vi "GEA3_Tool (Main).vi"() -> ()   [LabVIEW 2021]
panel:
  in  "Numeric":u64 format="%x"
  out "substring":string
  in  "dato":string="F039"
  in  "Write":bool
  in  "Read":bool
  in  "stop":bool
  out "CompleteFrame":string
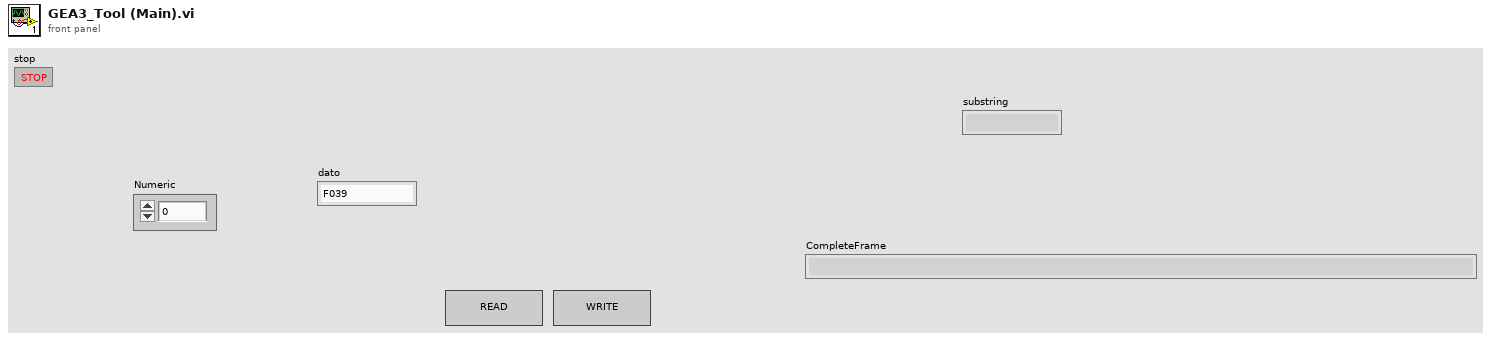
[diagram p1: front panel]
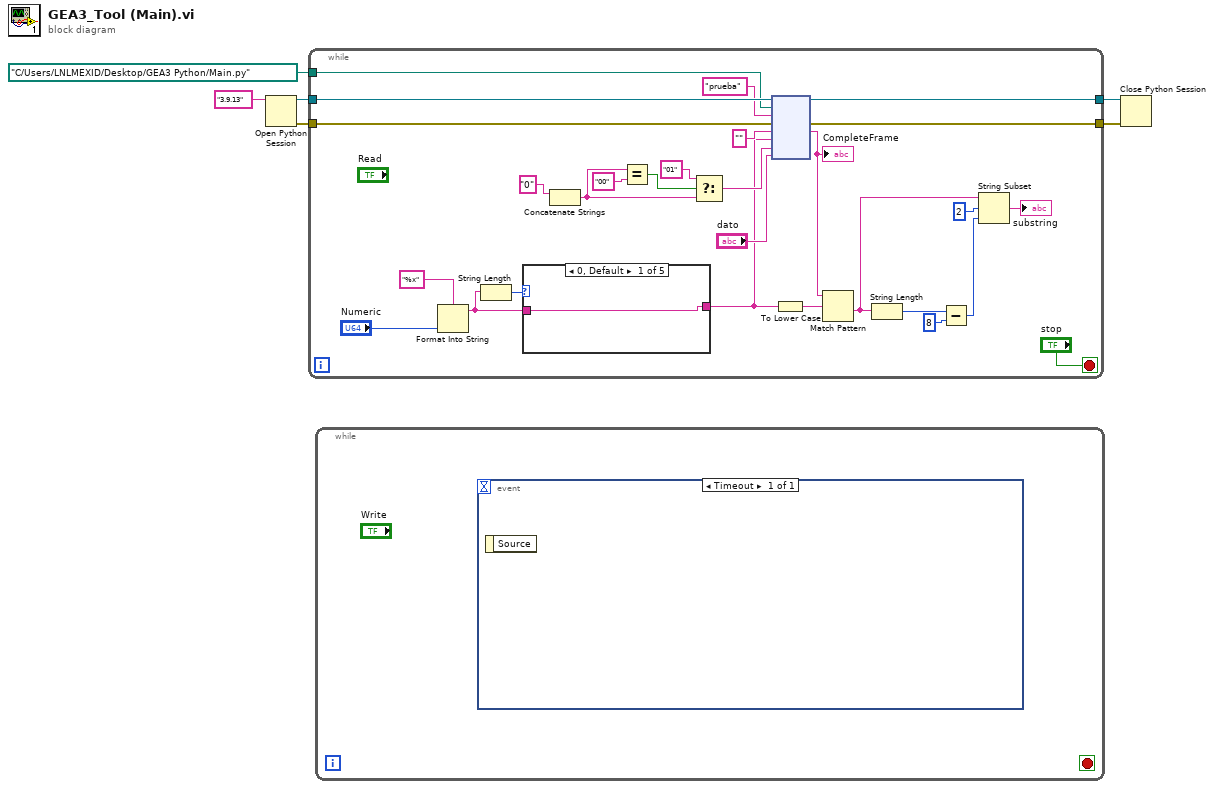
[diagram p0: block diagram]
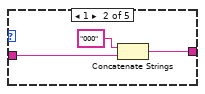
[diagram p2: hidden frame]
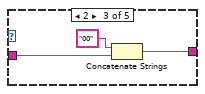
[diagram p3: hidden frame]
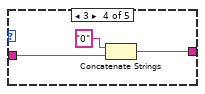
[diagram p4: hidden frame]
diagram:
  n1 = Open Python Session(python version="3.9.13" ("Python version")) -> (session out=w5:refnum<k35>, error out=w4:errorcluster)  [unwired: 2 in]
  n2 = while {
    tunnel: w5 -> [w34]
    tunnel: w4 -> [w33]
    tunnel: [w31] -> w3
    tunnel: [w30] -> w2
    tunnel: path "C:/Users/LNLMEXID/Desktop/GEA3 Python/Main.py" ("module path") -> [w13]
    stop <- "stop" stop-if-true
    n3 = Format Into String(format string="%x", "Numeric") -> (resulting string=w10:string)  [unwired: 2 in, 1 out]
    n4 = String Length(string=w10) -> (length=w12:i32)
    n5 = case shown="0, Default" w12 {
      tunnel: w10 -> [w35 w37 w40 w43 w45]
      tunnel: [w35 w36 w39 w42 w45] -> w8
      frame 0, Default {
      }
      frame 1 {
        n6 = Concatenate Strings("000" ("string"), w37) -> (w36:string)
      }
      frame 2 {
        n7 = Concatenate Strings("00" ("string"), w40) -> (w39:string)
      }
      frame 3 {
        n8 = Concatenate Strings("0" ("string"), w43) -> (w42:string)
      }
      frame 4 {
      }
    }
    n9 = Concatenate Strings("0" ("string")) -> (w22:string)  [unwired: 1 in]
    n10 = Equal?(x=w22, y="00") -> (x = y?=w24:bool)
    n11 = Select(t="01", s=w24, f=w22) -> (s? t:f=w21:string)
    n12 = node(w34, w13, "prueba" ("function name"), w33, "" ("data_hex"), w8, w21, "dato") -> (w31:refnum<k35>, w30:errorcluster, w20:string)  [unwired: 3 in, 2 out]
    "CompleteFrame" <- w20
    n13 = To Lower Case(string=w8) -> (all lower case string=w7:string)
    n14 = Match Pattern(string=w20, regular expression=w7) -> (after substring=w16:string)  [unwired: 1 in, 3 out]
    n15 = String Length(string=w16) -> (length=w19:i32)
    n16 = Subtract(x=w19, y=8) -> (x-y=w17:i32)
    n17 = String Subset(string=w16, offset (0)=2, length (rest)=w17) -> (substring=→"substring":string)
  }
  n18 = while {
    stop <- _ stop-if-true
    n19 = event shown="[0] Timeout" {
      selector: _ -> [_]
      dyn-events: _ -> [_]
      timeout: _ -> [_]
      event Timeout {
        n20 = event-data() -> ()  [unwired: 1 in, 1 out]
      }
    }
  }
  n21 = Close Python Session(session in=w3, error in=w2) -> ()  [unwired: 1 out]
